vi "Start_USB_DAQ.vi"(2 "USB ADDRESS In":i32=4660 format="%x", 3 "App Path":path) -> (0 "Abort":bool, 1 "USB ADDRESS 0ut":i32=4660 format="%x")   [LabVIEW 2011]
doc: "1. Checks to see if any USB-DAQ's are connected.\n2. If one or more USB-DAQ's is connected, it checks to see if the input USB address matches the address of the connected one of the USB devices. \n3. If the USB addresses matches, the VI exists with no error.\n4. If the USB address does not match, the VI brings up a window to let you select the correct device.\n5. If no device is detected, the software tells the user to check the hardware."
panel:
  # "Inputs"
  # "Outputs"
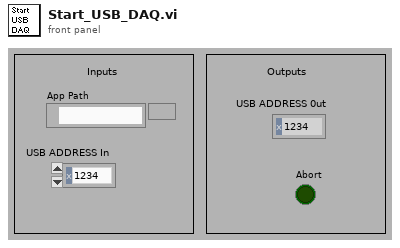
[diagram p1: front panel]
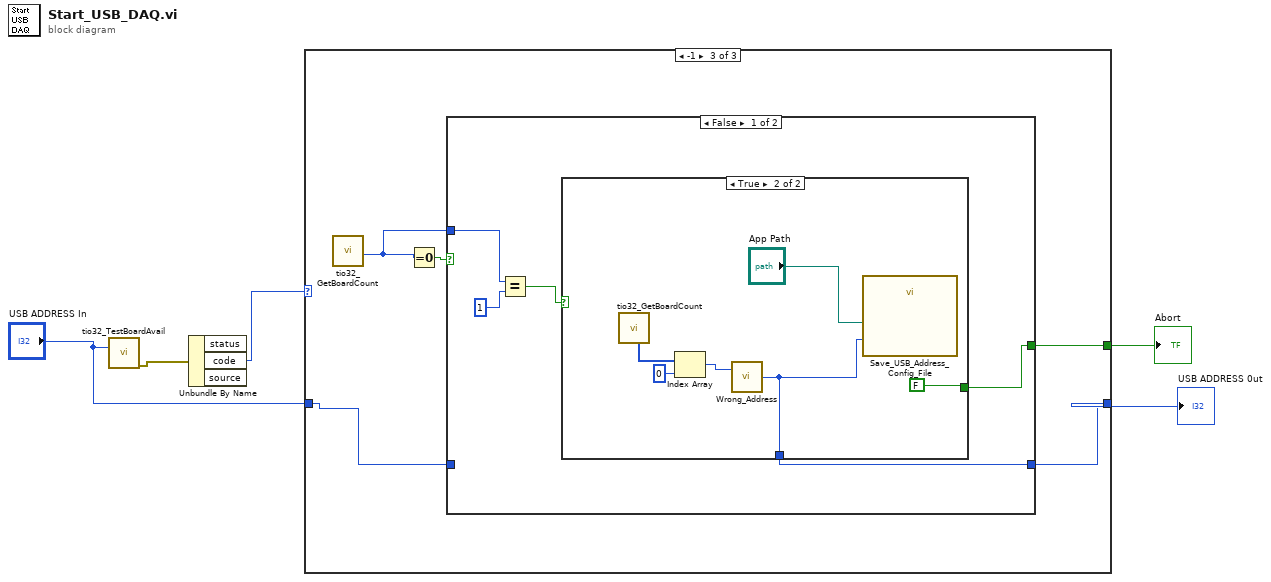
[diagram p0: block diagram]
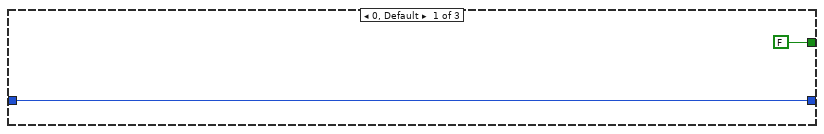
[diagram p2: hidden frame]
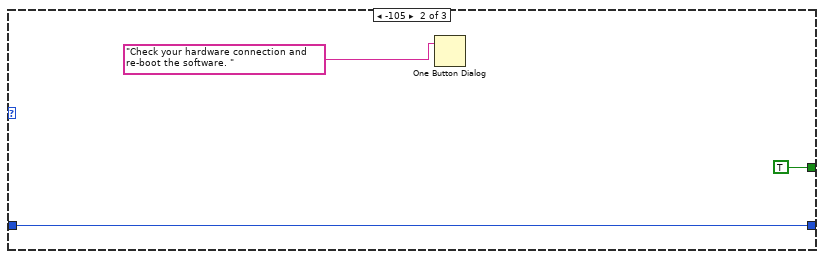
[diagram p3: hidden frame]
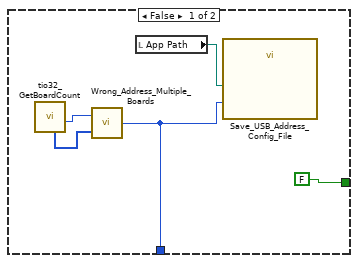
[diagram p4: hidden frame]
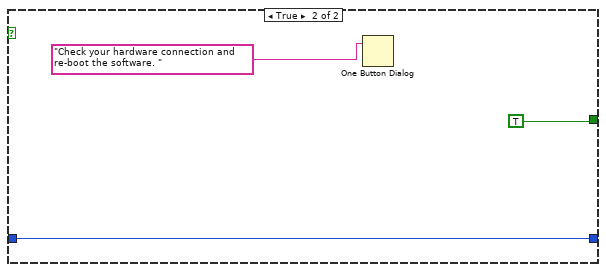
[diagram p5: hidden frame]
diagram:
  n1 = call "tio32_TestBoardAvail.vi"("device addess to check"="USB ADDRESS In") -> ("error out"=w4:errorcluster)  [unwired: 11 in, 3 out]
  n2 = Unbundle By Name(w4) -> ("code"=w5:i32)  [unwired: 2 out]
  n3 = case shown="-1" w5 {
    tunnel: [w7 w10 w13] -> w3
    tunnel: "USB ADDRESS In" -> [w7 w10 w12]
    tunnel: [FALSE TRUE w11] -> w1
    frame 0, Default {
    }
    frame -105 {
      n4 = One Button Dialog(message="Check your hardware connection and re-boot the software. " ("error source (\" \")")) -> ()  [unwired: 1 in, 1 out]
    }
    frame -1 {
      n5 = call "tio32_GetBoardCount.vi"() -> ("# of boards"=w15:i32)  [unwired: 7 in, 4 out]
      n6 = Equal To 0?(x=w15) -> (x = 0?=w14:bool)
      n7 = case shown="False" w14 {
        tunnel: w15 -> [w20 _]
        tunnel: [w18 w34] -> w13
        tunnel: w12 -> [_ w34]
        tunnel: [w16 TRUE] -> w11
        frame False {
          n8 = Equal?(x=w20, y=1 ("x")) -> (x = y?=w17:bool)
          n9 = case shown="True" w17 {
            tunnel: [w23 w28] -> w18
            tunnel: [FALSE FALSE] -> w16
            frame False {
              n10 = call "tio32_GetBoardCount.vi"() -> ("# of boards"=w24:i32, "Address"=w25:i32[])  [unwired: 7 in, 3 out]
              n11 = call "Wrong_Address_Multiple_Boards.vi"("In Addresses available"=w25, "numb boards"=w24) -> ("New Address"=w23:i32)
              n12 = local read "App Path"() -> (w22:path)
              n13 = call "Save_USB_Address_Config_File.vi"("App Path"=w22, "USB DAQ Address"=w23) -> ()
            }
            frame True {
              n14 = call "tio32_GetBoardCount.vi"() -> ("Address"=w29:i32[])  [unwired: 7 in, 4 out]
              n15 = Index Array(array=w29, index=0) -> (element=w30:i32)
              n16 = call "Wrong_Address.vi"("Hardware Address"=w30) -> ("New Software Address"=w28:i32)  [unwired: 1 in]
              n17 = call "Save_USB_Address_Config_File.vi"("App Path"="App Path", "USB DAQ Address"=w28) -> ()
            }
          }
        }
        frame True {
          n18 = One Button Dialog(message="Check your hardware connection and re-boot the software. " ("error source (\" \")")) -> ()  [unwired: 1 in, 1 out]
        }
      }
    }
  }
  "USB ADDRESS 0ut" <- w3
  "Abort" <- w1
